vi "Remove Publisher Instance Command.vi"(8 "error in":errorcluster, 10 "Publisher Name":string, 11 "CIFCorePlugin in":refnum<class "CIFCorePlugin.lvclass">) -> (0 "error out":errorcluster, 3 "CIFCorePlugin out":refnum<class "CIFCorePlugin.lvclass">)   [LabVIEW 2021, in "CIFCorePlugin.lvclass"]
uses:
  CIFCorePlugin.lvclass
  Typedef/gRPC to Main Commands.ctl
  7097a809-caa9-496b-b674-de659a984328.vi
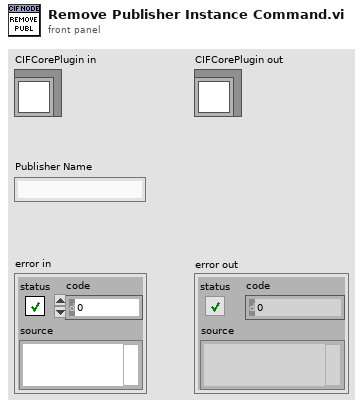
[diagram p1: front panel]
types:
  T1 = typedef "CIFCorePlugin.lvclass/gRPC to Main Commands.ctl" = enum8{"Start", "Pause", "Stop", "RefreshStats", "UpdateConfig", "Update Clock Map", "Connect Channel", "Force Channel", "Add Publisher Instance", "Remove Publisher Instance"}
  T2 = typedef "CIFCorePlugin.lvclass/gRPC to Main DVR.ctl" = refnum<data-value>
  T3 = typedef "CIFCoreCommon.lvlib/gRPC to Main Data.ctl" = cluster{"Config Data":variant, "Connection":T4, "Force":T5, "Clock Conversion":T6, "Publisher Instance":T8}
  T4 = typedef "CIFCoreCommon.lvlib/Channel Connection Data.ctl" = cluster{"Publisher Name":string, "Subscriber Name":string, "Connection Data":u8[]}
  T5 = typedef "CIFCoreCommon.lvlib/Channel Force Data.ctl" = cluster{"Channel Name":string, "Force Data":u8[], "Force Active":bool}
  T6 = typedef "Time_CIF_U.lvlib/Clock Conversion Map.ctl" = map{u8, cluster{"Last Reset":i64, "Offset Pair":T7, "Slope":dbl, "1/Slope":dbl}}
  T7 = typedef "Time_CIF_U.lvlib/Timestamp Pair.ctl" = cluster{"System Time":i64, "External Time":i64}
  T8 = typedef "CIFCoreCommon.lvlib/FIFO Publisher.ctl" = cluster{"Publisher Name":string, "New FIFO Instance Config":T9}
  T9 = typedef "ChannelCommon.lvlib/New FIFO Instance Configuration.ctl" = cluster{"Primary":bool, "Backpressure":bool, "Message/FIFO Override":u32}
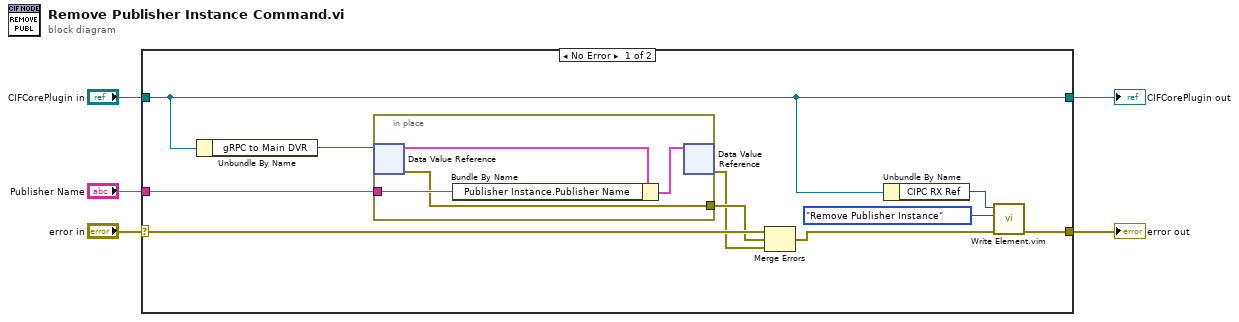
[diagram p0: block diagram]
diagram:
  n1 = case shown="No Error" "error in" {
    selector: "error in" -> [w9 w21]
    tunnel: [w14 w21] -> w4
    tunnel: "CIFCorePlugin in" -> [w12 w20]
    tunnel: [w12 w20] -> w2
    tunnel: "Publisher Name" -> [w10 _]
    frame No Error {
      n2 = Unbundle By Name(w12) -> ("gRPC to Main DVR"=w11:T2)
      n3 = in-place {
        in-place-border: w10 -> [w17]
        in-place-border: [w16] -> w8
        n4 = in-place-dvr #1(w11) -> (w19:T3, w16:errorcluster)
        n5 = Bundle By Name(cluster=w19, "Publisher Instance.Publisher Name"=w17) -> (w18:T3)
        n6 = in-place-dvr #1(w18) -> (w7:errorcluster)  [unwired: 1 out]
      }
      n7 = Merge Errors(w9, w8, w7) -> (w6:errorcluster)
      n8 = Unbundle By Name(w12) -> ("CIPC RX Ref"=w13:u64)
      n9 = call "Write Element.vim"("error in (no error)"=w6, "Data in"=gRPC_to_Main_Commands."Remove Publisher Instance" ("OOB Main Commands"), "CIPC Reference in"=w13) -> ("error out"=w14:errorcluster)  [unwired: 5 in, 3 out]
    }
    frame Error {
    }
  }
  "error out" <- w4
  "CIFCorePlugin out" <- w2
